vi "题目7.vi"() -> ()   [LabVIEW 2017]
uses:
  <vilib>/Utility/file.llb/Read Delimited Spreadsheet (DBL).vi
  <vilib>/Analysis/NI_AALBase.lvlib
panel:
  out "all rows":dbl[][](array[numeric]) caption="所有行"
  in  "cycles":dbl=1.0 caption="周期" format="%0.2f"
  out "拆分的路径":path
  out "波形图":dbl[](graph)
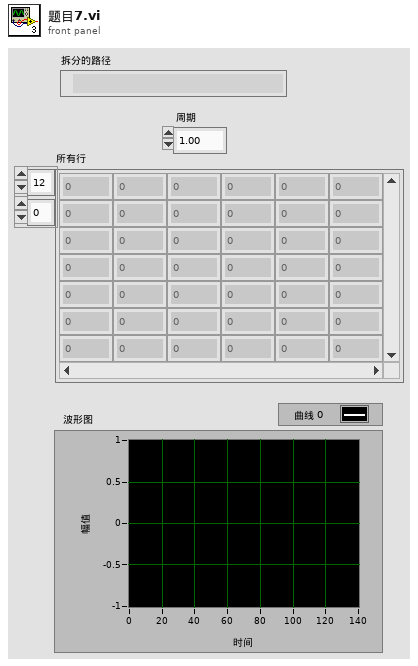
[diagram p1: front panel]
types:
  T1 = enum16{"open", "replace", "create", "open or create", "replace or create", "replace or create with confirmation"}
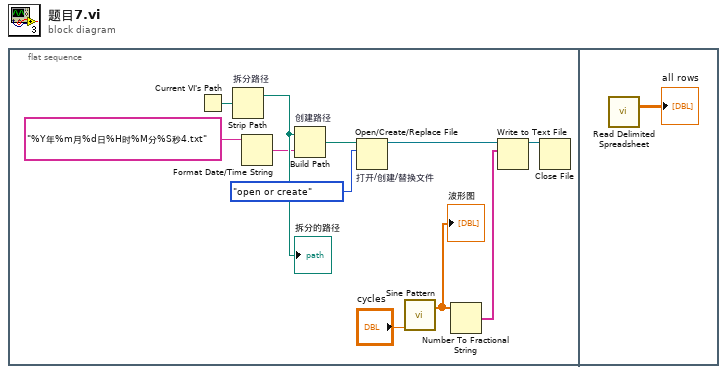
[diagram p0: block diagram]
diagram:
  n1 = flat-sequence {
    frame #0 {
      n2 = Current VI's Path() -> (path=w7:path)
      n3 = Strip Path "拆分路径"(path=w7) -> (stripped path=w8:path)  [unwired: 1 out]
      "拆分的路径" <- w8
      n4 = Format Date/Time String(time format string (%c)="%Y年%m月%d日%H时%M分%S秒4.txt" ("时间格式字符串(%c)")) -> (date/time string=w5:string)  [unwired: 2 in]
      n5 = Build Path "创建路径"(base path=w8, name or relative path=w5) -> (appended path=w2:path)
      n6 = Open/Create/Replace File "打开/创建/替换文件"(file path (use dialog)=w2, operation (0:open)=T1."open or create" ("操作(0:open)")) -> (refnum out=w4:refnum<file>)  [unwired: 4 in, 2 out]
      n7 = call <vilib>:"Sine Pattern.vi"("cycles"="cycles") -> ("Sinusoidal Pattern"=w1:dbl[])  [unwired: 3 in, 1 out]
      "波形图" <- w1
      n8 = Number To Fractional String(number=w1) -> (F-format string=w10:string[])  [unwired: 3 in]
      n9 = Write to Text File(file (use dialog)=w4, text=w10) -> (refnum out=w3:refnum<file>)  [unwired: 2 in, 2 out]
      n10 = Close File(refnum=w3) -> ()  [unwired: 1 in, 2 out]
    }
    frame #1 {
      n11 = call-poly <vilib>:"Read Delimited Spreadsheet.vi"() -> ("all rows"=→"all rows":dbl[][])  [unwired: 10 in, 5 out]
    }
  }
